vi "Instrument.DAQ Activity Tree.vi"   [LabVIEW 2019, in "Instrument.Lockin.lvlib" / "Instrument.DAQ.lvclass"]
uses:
  Instrument.DAQ.lvclass
types:
  T1 = typedef "Instrument.Lockin.lvlib/Instrument.DAQ.lvclass/PublicEvents--Cluster.ctl" = cluster{"getAIChannels":refnum<user-event>, "getAOChannels":refnum<user-event>, "getREFChannels":refnum<user-event>, "getWaveforms":refnum<user-event>, "getResults":refnum<user-event>, "getSweepWaveforms":refnum<user-event>, "getCalibration":refnum<user-event>, "getDAQState":refnum<user-event>, "getDAQconfig":refnum<user-event>, "getInputGain":refnum<user-event>, "getOutputGain":refnum<user-event>, "getInputOffset":refnum<user-event>, "getSampling":refnum<user-event>, "getSweepChannels":refnum<user-event>, "getDeviceIDN":refnum<user-event>}
  T2 = typedef "Instrument.Lockin.lvlib/Instrument.DAQ.lvclass/PrivateEvents--Cluster.ctl" = cluster{"setAOconfig":refnum<user-event>, "setAIconfig":refnum<user-event>, "setAO":refnum<user-event>, "setREF":refnum<user-event>, "setSampling":refnum<user-event>, "setState":refnum<user-event>, "setInputGain":refnum<user-event>, "setOutputGain":refnum<user-event>, "setSweep":refnum<user-event>, "measureOffset":refnum<user-event>, "zeroOffset":refnum<user-event>, "setPreFilter":refnum<user-event>, "autoConfigureDAQ":refnum<user-event>, "setCalibration":refnum<user-event>, "setAI":refnum<user-event>, "zeroPhase":refnum<user-event>, "setAmplitudeLimit":refnum<user-event>, "setLinkFrequencies":refnum<user-event>, "showUI":refnum<user-event>, "setInputOffset":refnum<user-event>, "setDCLimit":refnum<user-event>, "setDutyCycle":refnum<user-event>}
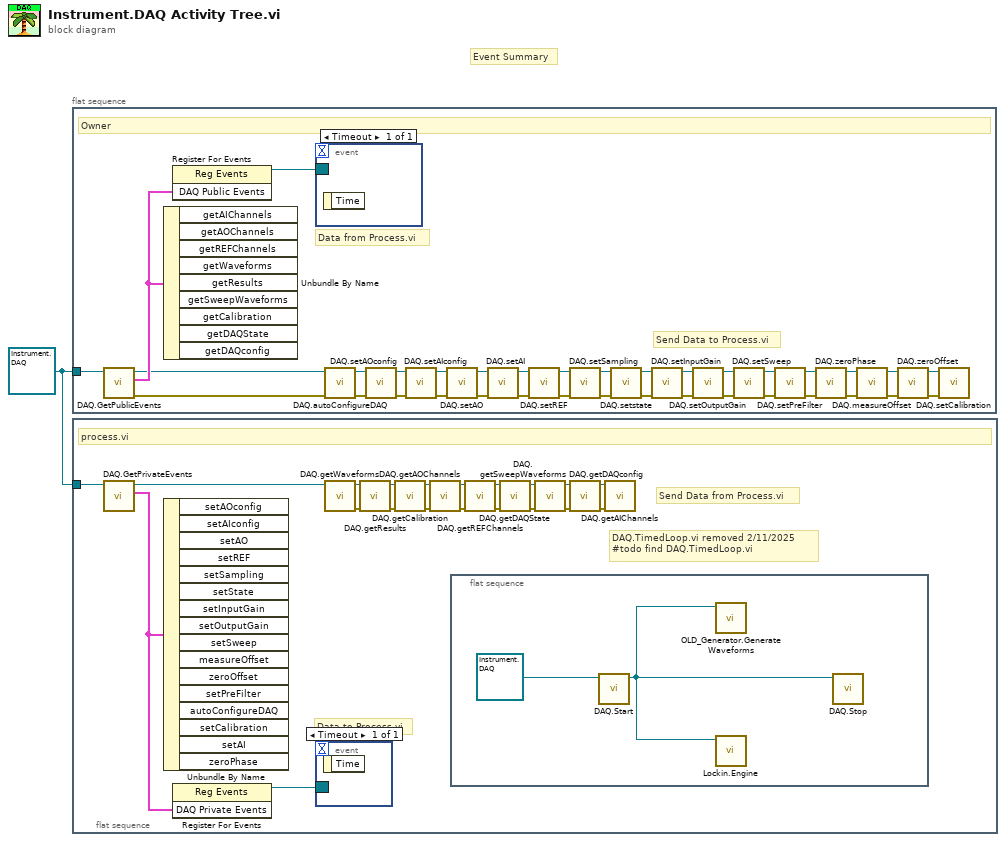
[diagram p0: block diagram]
diagram:
  w1 = refnum<class "Instrument.DAQ.lvclass"> refnum ("Instrument.DAQ.lvclass")
  # "Event Summary"
  n1 = flat-sequence {
    tunnel: w1 -> [w36]
    frame #0 {
      # "Data from Process.vi"
      # "Send Data to Process.vi"
      # "Owner"
      n2 = call "DAQ.GetPublicEvents.vi"("Instrument.DAQ"=w36) -> ("error out"=w32:errorcluster, "DAQ Public Events"=w34:T1, "Instrument.DAQ out"=w33:refnum<class "Instrument.DAQ.lvclass">)  [unwired: 8 in]
      n3 = Unbundle By Name(w34) -> ()  [unwired: 9 out]
      n4 = register-events(w34) -> (reference out=w35:refnum<event-registration>)  [unwired: 2 in, 1 out]
      n5 = event shown="[0] Timeout" {
        selector: w35 -> [_]
        dyn-events: _ -> [_]
        timeout: _ -> [_]
        event Timeout {
          n6 = event-data() -> ()  [unwired: 1 in, 1 out]
        }
      }
      n7 = call "DAQ.autoConfigureDAQ.vi"("error in (no error)"=w32, "Instrument.DAQ"=w33) -> ("error out"=w30:errorcluster, "Instrument.DAQ out"=w31:refnum<class "Instrument.DAQ.lvclass">)  [unwired: 8 in]
      n8 = call "DAQ.setAOconfig.vi"("error in (no error)"=w30, "Instrument.DAQ"=w31) -> ("error out"=w28:errorcluster, "Instrument.DAQ out"=w29:refnum<class "Instrument.DAQ.lvclass">)  [unwired: 8 in]
      n9 = call "DAQ.setAIconfig.vi"("error in (no error)"=w28, "Instrument.DAQ"=w29) -> ("error out"=w26:errorcluster, "Instrument.DAQ out"=w27:refnum<class "Instrument.DAQ.lvclass">)  [unwired: 8 in]
      n10 = call "DAQ.setAO.vi"("error in (no error)"=w26, "Instrument.DAQ"=w27) -> ("error out"=w24:errorcluster, "Instrument.DAQ out"=w25:refnum<class "Instrument.DAQ.lvclass">)  [unwired: 8 in]
      n11 = call "DAQ.setAI.vi"("error in (no error)"=w24, "Instrument.DAQ"=w25) -> ("error out"=w22:errorcluster, "Instrument.DAQ out"=w23:refnum<class "Instrument.DAQ.lvclass">)  [unwired: 8 in]
      n12 = call "DAQ.setREF.vi"("error in (no error)"=w22, "Instrument.DAQ"=w23) -> ("error out"=w20:errorcluster, "Instrument.DAQ out"=w21:refnum<class "Instrument.DAQ.lvclass">)  [unwired: 8 in]
      n13 = call "DAQ.setSampling.vi"("error in (no error)"=w20, "Instrument.DAQ"=w21) -> ("error out"=w18:errorcluster, "Instrument.DAQ out"=w19:refnum<class "Instrument.DAQ.lvclass">)  [unwired: 8 in]
      n14 = call "DAQ.setstate.vi"("error in (no error)"=w18, "Instrument.DAQ"=w19) -> ("error out"=w16:errorcluster, "Instrument.DAQ out"=w17:refnum<class "Instrument.DAQ.lvclass">)  [unwired: 8 in]
      n15 = call "DAQ.setInputGain.vi"("error in (no error)"=w16, "Instrument.DAQ"=w17) -> ("error out"=w14:errorcluster, "Instrument.DAQ out"=w15:refnum<class "Instrument.DAQ.lvclass">)  [unwired: 8 in]
      n16 = call "DAQ.setOutputGain.vi"("error in (no error)"=w14, "Instrument.DAQ"=w15) -> ("error out"=w12:errorcluster, "Instrument.DAQ out"=w13:refnum<class "Instrument.DAQ.lvclass">)  [unwired: 8 in]
      n17 = call "DAQ.setSweep.vi"("error in (no error)"=w12, "Instrument.DAQ"=w13) -> ("error out"=w10:errorcluster, "Instrument.DAQ out"=w11:refnum<class "Instrument.DAQ.lvclass">)  [unwired: 8 in]
      n18 = call "DAQ.setPreFilter.vi"("error in (no error)"=w10, "Instrument.DAQ"=w11) -> ("error out"=w8:errorcluster, "Instrument.DAQ out"=w9:refnum<class "Instrument.DAQ.lvclass">)  [unwired: 8 in]
      n19 = call "DAQ.zeroPhase.vi"("error in (no error)"=w8, "Instrument.DAQ"=w9) -> ("error out"=w6:errorcluster, "Instrument.DAQ out"=w7:refnum<class "Instrument.DAQ.lvclass">)  [unwired: 8 in]
      n20 = call "DAQ.measureOffset.vi"("error in (no error)"=w6, "Instrument.DAQ"=w7) -> ("error out"=w4:errorcluster, "Instrument.DAQ out"=w5:refnum<class "Instrument.DAQ.lvclass">)  [unwired: 8 in]
      n21 = call "DAQ.zeroOffset.vi"("error in (no error)"=w4, "Instrument.DAQ"=w5) -> ("error out"=w2:errorcluster, "Instrument.DAQ out"=w3:refnum<class "Instrument.DAQ.lvclass">)  [unwired: 8 in]
      n22 = call "DAQ.setCalibration.vi"("error in (no error)"=w2, "Instrument.DAQ"=w3) -> ()  [unwired: 8 in, 2 out]
    }
  }
  n23 = flat-sequence {
    tunnel: w1 -> [w56]
    frame #0 {
      # "DAQ.TimedLoop.vi removed 2/11/2025\n#todo find DAQ.TimedLoop.vi"
      # "Data to Process.vi"
      # "Send Data from Process.vi"
      # "process.vi"
      n24 = call "DAQ.GetPrivateEvents.vi"("Instrument.DAQ"=w56) -> ("DAQ Private Events"=w55:T2, "Instrument.DAQ"=w40:refnum<class "Instrument.DAQ.lvclass">)  [unwired: 8 in, 1 out]
      n25 = Unbundle By Name(w55) -> ()  [unwired: 16 out]
      n26 = register-events(w55) -> (reference out=w39:refnum<event-registration>)  [unwired: 2 in, 1 out]
      n27 = event shown="[0] Timeout" {
        selector: w39 -> [_]
        dyn-events: _ -> [_]
        timeout: _ -> [_]
        event Timeout {
          n28 = event-data() -> ()  [unwired: 1 in, 1 out]
        }
      }
      n29 = call "DAQ.getWaveforms.vi"("Instrument.DAQ"=w40) -> ("error out"=w53:errorcluster, "Instrument.DAQ"=w54:refnum<class "Instrument.DAQ.lvclass">)  [unwired: 9 in]
      n30 = call "DAQ.getResults.vi"("error in (no error)"=w53, "Instrument.DAQ"=w54) -> ("error out"=w51:errorcluster, "Instrument.DAQ out"=w52:refnum<class "Instrument.DAQ.lvclass">)  [unwired: 8 in]
      n31 = call "DAQ.getCalibration.vi"("error in (no error)"=w51, "Instrument.DAQ"=w52) -> ("error out"=w49:errorcluster, "Instrument.DAQ"=w50:refnum<class "Instrument.DAQ.lvclass">)  [unwired: 8 in]
      n32 = call "DAQ.getAOChannels.vi"("error in (no error)"=w49, "Instrument.DAQ"=w50) -> ("error out"=w47:errorcluster, "Instrument.DAQ out"=w48:refnum<class "Instrument.DAQ.lvclass">)  [unwired: 8 in]
      n33 = flat-sequence {
        frame #0 {
          n34 = call "DAQ.Start.vi"("Instrument.DAQ"=refnum<class "Instrument.DAQ.lvclass"> refnum) -> ("Instrument.DAQ out"=w58:refnum<class "Instrument.DAQ.lvclass">)  [unwired: 9 in, 1 out]
          n35 = call "OLD_Generator.Generate Waveforms.vi"("Instrument.DAQ"=w58) -> ()  [unwired: 8 in, 3 out]
          n36 = call "Lockin.Engine.vi"("Instrument.DAQ"=w58) -> ()  [unwired: 6 in, 5 out]
          n37 = call "DAQ.Stop.vi"("Instrument.DAQ in"=w58) -> ()  [unwired: 9 in, 2 out]
        }
      }
      n38 = call "DAQ.getREFChannels.vi"("error in (no error)"=w47, "Instrument.DAQ"=w48) -> ("error out"=w45:errorcluster, "Instrument.DAQ out"=w46:refnum<class "Instrument.DAQ.lvclass">)  [unwired: 8 in]
      n39 = call "DAQ.getDAQState.vi"("error in (no error)"=w45, "Instrument.DAQ"=w46) -> ("error out"=w43:errorcluster, "Instrument.DAQ out"=w44:refnum<class "Instrument.DAQ.lvclass">)  [unwired: 8 in]
      n40 = call "DAQ.getSweepWaveforms.vi"("error in (no error)"=w43, "Instrument.DAQ"=w44) -> ("error out"=w41:errorcluster, "Instrument.DAQ out"=w42:refnum<class "Instrument.DAQ.lvclass">)  [unwired: 8 in]
      n41 = call "DAQ.getDAQconfig.vi"("error in (no error)"=w41, "Instrument.DAQ"=w42) -> ("error out"=w37:errorcluster, "Instrument.DAQ out"=w38:refnum<class "Instrument.DAQ.lvclass">)  [unwired: 8 in]
      n42 = call "DAQ.getAIChannels.vi"("error in (no error)"=w37, "Instrument.DAQ"=w38) -> ()  [unwired: 8 in, 2 out]
    }
  }
